vi "createActionEvent.vi"(8 "error in (no error)":errorcluster, 11 "QControl_Graph in":refnum<class "QControl_Graph.lvclass">) -> (0 "error out":errorcluster, 3 "QControl_Graph out":refnum<class "QControl_Graph.lvclass">)   [LabVIEW 2017, in "QControl_Graph.lvclass"]
uses:
  QControl_Graph.lvclass
  QControl_Graph.lvclass/QControl_Graph.ctl
  Actions.ctl
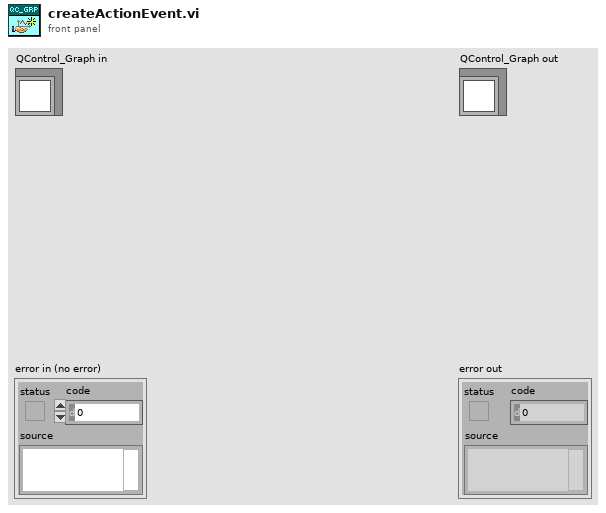
[diagram p1: front panel]
types:
  T1 = typedef "QControl_Graph.lvclass/Actions.ctl" = enum16{"Undefined", "BGK Color", "Highlight Plot", "Mouse Zoom", "Show Cursors", "Show Markers"}
  T2 = typedef "QControl_Graph.lvclass/State Data.ctl" = cluster{"Data":bool, "Action Performed":refnum<user-event>}
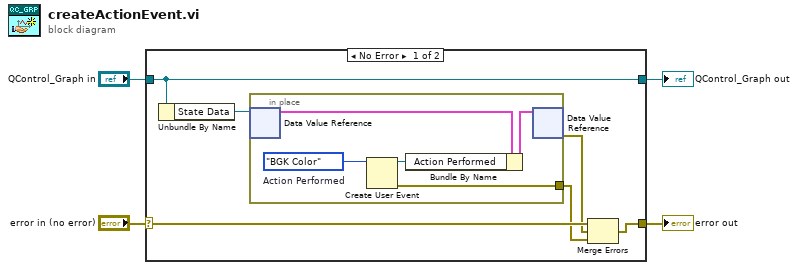
[diagram p0: block diagram]
diagram:
  n1 = case shown="No Error" "error in (no error)" {
    selector: "error in (no error)" -> [w10 w17]
    tunnel: [w7 w17] -> w3
    tunnel: [w9 w16] -> w1
    tunnel: "QControl_Graph in" -> [w9 w16]
    frame No Error {
      n2 = Unbundle By Name(w9) -> ("State Data"=w8:refnum<data-value>)
      n3 = in-place {
        in-place-border: [w15] -> w5
        w14 = Actions."BGK Color"  # Action Performed
        n4 = in-place-dvr #1(w8) -> (w13:T2)  [unwired: 1 out]
        n5 = Create User Event(user event datatype=w14) -> (user event=w11:refnum<user-event>, error out=w15:errorcluster)  [unwired: 1 in]
        n6 = Bundle By Name(cluster=w13, "Action Performed"=w11) -> (w12:T2)
        n7 = in-place-dvr #1(w12) -> (w6:errorcluster)  [unwired: 1 out]
      }
      n8 = Merge Errors(w10, w6, w5) -> (w7:errorcluster)
    }
    frame Error {
    }
  }
  "error out" <- w3
  "QControl_Graph out" <- w1
